vi "Exp_ICCD_GetOnChipAccumulations.vi"(8 "error in (no error)":errorcluster, 11 "LightField Automation in":refnum<class "LightField Automation.lvclass">) -> (0 "error out":errorcluster, 2 "On Chip Accumulations":i32, 3 "LightField Automation out":refnum<class "LightField Automation.lvclass">)   [LabVIEW 2013, in "LightField Automation.lvclass"]
uses:
  LightField Automation.lvclass
  C:/Program Files/Princeton Instruments/LightField/PrincetonInstruments.LightFieldAddInSupportServices.dll
  Program Files/Princeton Instruments/LightField/PrincetonInstruments.LightFieldAddInSupportServices.dll
  LightField Automation.lvclass/LightField Automation.ctl
  C:/Program Files/Princeton Instruments/LightField/AddInViews/PrincetonInstruments.LightFieldViewV3.dll
  Program Files/Princeton Instruments/LightField/AddInViews/PrincetonInstruments.LightFieldViewV3.dll
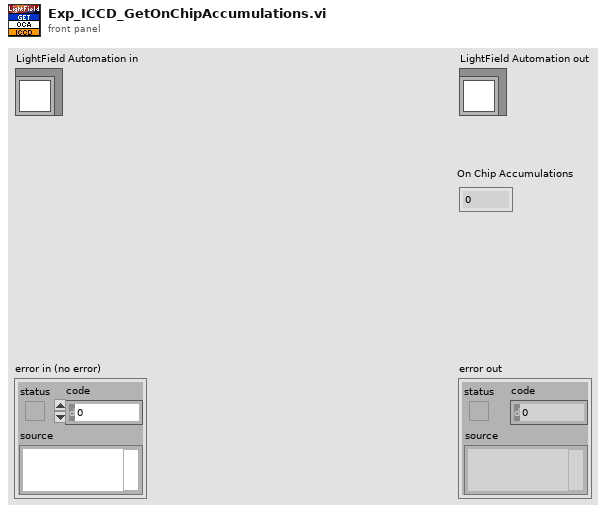
[diagram p1: front panel]
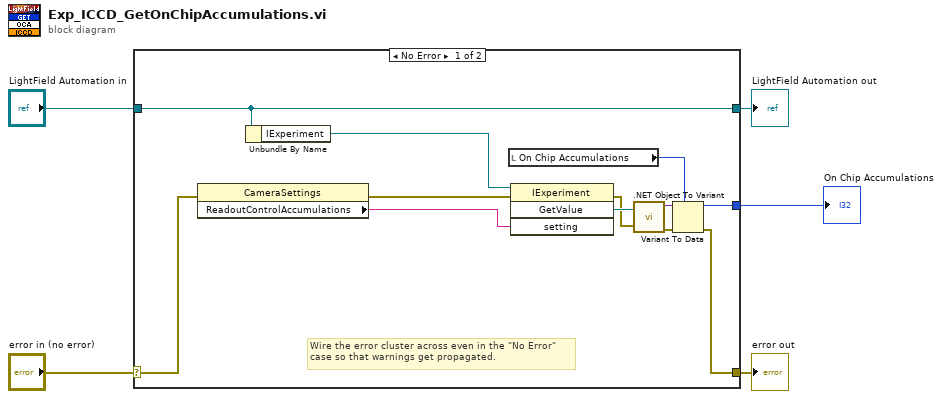
[diagram p0: block diagram]
diagram:
  n1 = case shown="No Error" "error in (no error)" {
    selector: "error in (no error)" -> [w8 w19]
    tunnel: [w10 w19] -> w4
    tunnel: [w13 w18] -> w2
    tunnel: "LightField Automation in" -> [w13 w18]
    tunnel: [w11 _] -> w1
    frame No Error {
      # "Wire the error cluster across even in the \"No Error\"\ncase so that warnings get propagated."
      n2 = property class="CameraSettings"(error in=w8) -> (error out=w6:errorcluster, "ReadoutControlAccumulations"=w7:string)  [unwired: 1 in, 1 out]
      n3 = Unbundle By Name(w13) -> ("IExperiment"=w12:refnum<k24>)
      n4 = local read "On Chip Accumulations"() -> (w9:i32)
      n5 = invoke class="IExperiment" method="GetValue"(reference=w12, error in=w6, "setting"=w7) -> (error out=w14:errorcluster, "GetValue"=w15:refnum<k24>)  [unwired: 1 in, 2 out]
      n6 = call <vilib>:".NET Object To Variant.vi"("error in (no error)"=w14, ".NET object"=w15) -> ("error out"=w17:errorcluster, "variant"=w16:variant)
      n7 = Variant To Data(error in=w17, type=w9, Variant=w16) -> (data=w11:i32, error out=w10:errorcluster)
    }
    frame Error {
    }
  }
  "error out" <- w4
  "LightField Automation out" <- w2
  "On Chip Accumulations" <- w1
